vi "Strip brackets.vi"(3 "trimmed string in":string) -> (0 "trimmed string out":string)   [LabVIEW 2017]
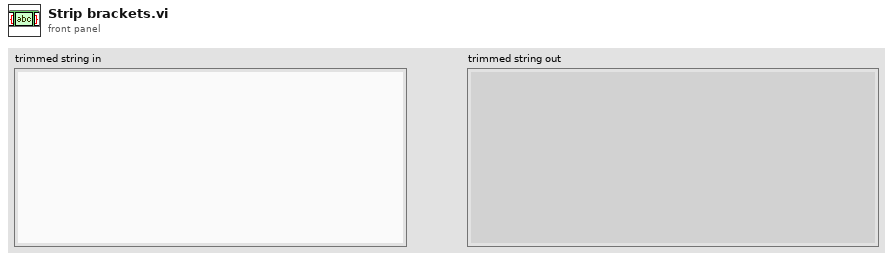
[diagram p1: front panel]
types:
  T1 = enum16{"0x2829 - ()", "0x5B5D - []", "0x7B7D - {}"}
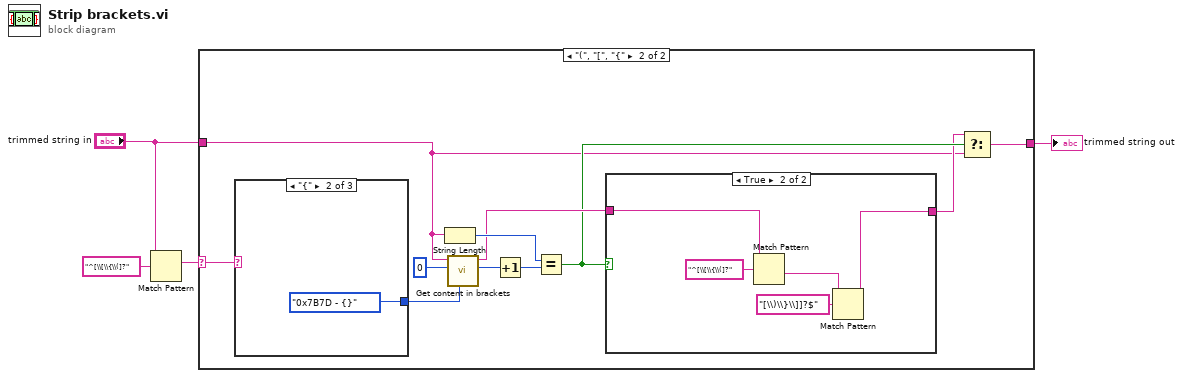
[diagram p0: block diagram]
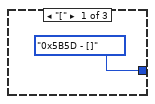
[diagram p4: hidden frame]
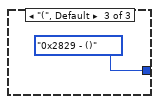
[diagram p5: hidden frame]
diagram:
  n1 = Match Pattern(string="trimmed string in", regular expression="^[\\[\\{\\(]?") -> (match substring=w2:string)  [unwired: 1 in, 3 out]
  n2 = case shown="\"(\", \"[\", \"{\"" w2 {
    selector: w2 -> [_ w16]
    tunnel: [w5 w10] -> w4
    tunnel: "trimmed string in" -> [w5 w7]
    frame "", Default {
    }
    frame "(", "[", "{" {
      n3 = case shown="\"{\"" w16 {
        tunnel: [T1."0x5B5D - []" ("TYPE") T1."0x7B7D - {}" ("TYPE") T1."0x2829 - ()" ("TYPE")] -> w6
        frame "[" {
        }
        frame "{" {
        }
        frame "(", Default {
        }
      }
      n4 = String Length(string=w7) -> (length=w13:i32)
      n5 = call "Get content in brackets.vi"("TYPE"=w6, "start"=0, "String in"=w7) -> ("index out"=w14:i32, "String out"=w12:string)  [unwired: 7 in]
      n6 = Increment(x=w14) -> (x+1=w11:i32)
      n7 = Equal?(x=w13, y=w11) -> (x = y?=w9:bool)
      n8 = case shown="True" w9 {
        tunnel: [w17 w22] -> w8
        tunnel: w12 -> [w17 w20]
        frame False {
        }
        frame True {
          n9 = Match Pattern(string=w20, regular expression="^[\\[\\{\\(]?") -> (after substring=w19:string)  [unwired: 1 in, 3 out]
          n10 = Match Pattern(string=w19, regular expression="[\\)\\}\\]]?$") -> (before substring=w22:string)  [unwired: 1 in, 3 out]
        }
      }
      n11 = Select(t=w8, s=w9, f=w7) -> (s? t:f=w10:string)
    }
  }
  "trimmed string out" <- w4
